vi "Start Point.vi"(5 "Series Enqueuer":refnum<class "Message Enqueuer.lvclass">, 7 "Task-Point Ident":string, 8 "error in":errorcluster, 11 "MSS in":refnum<class "MSS.lvclass">) -> (0 "error out":errorcluster, 3 "MSS out":refnum<class "MSS.lvclass">)   [LabVIEW 2023, in "HAL.lvlib" / "MSS.lvclass"]
uses:
  MSS.lvclass
  <vilib>/ActorFramework/Message Enqueuer/Message Enqueuer.lvclass
  MSS.lvclass/MSS.ctl
  MAL/Series/ISeries Actor/ISeries Actor Messages/Log Event Msg/Log Event Msg.lvclass/Log Event Msg.ctl
  <vilib>/ActorFramework/Message Enqueuer/Message Enqueuer.lvclass/Message Enqueuer.ctl
  MAL/Series/ISeries Actor/ISeries Actor Messages/Start Point on Target Msg/Start Point on Target Msg.lvclass/Start Point on Target Msg.ctl
  <vilib>/ActorFramework/Message Enqueuer/Enqueue.vi
  MAL/Series/ISeries Actor/ISeries Actor Messages/Log Event Msg/Log Event Msg.lvclass
  MAL/Series/ISeries Actor/ISeries Actor Messages/Start Point on Target Msg/Start Point on Target Msg.lvclass
  <vilib>/Utility/LVClass/Get LV Class Name.vi
  <resource>/AFDebug/Generate Trace for Message.vi
  <vilib>/ActorFramework/Message Priority Queue/Priority Enqueue.vi
  Virtual Instruments/Virtual Instrument/Virtual Instrument.lvclass
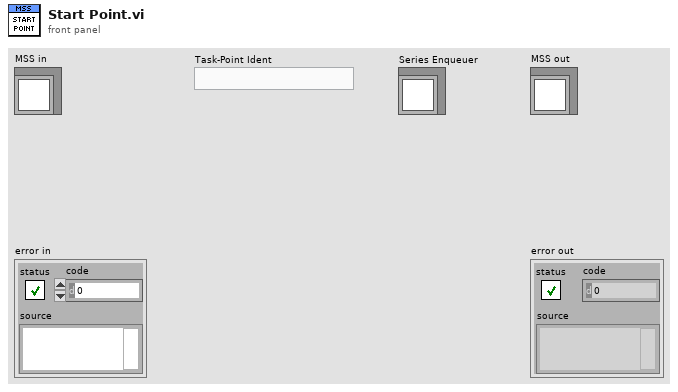
[diagram p1: front panel]
types:
  T1 = map{string, refnum<class "Virtual Instrument.lvclass">}
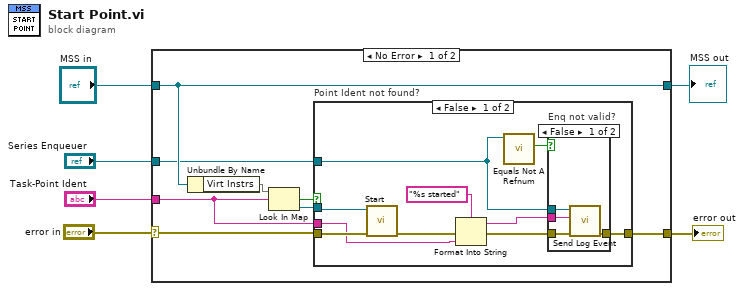
[diagram p0: block diagram]
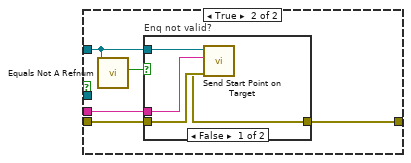
[diagram p3: hidden frame]
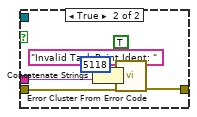
[diagram p4: hidden frame]
diagram:
  n1 = case shown="No Error" "error in" {
    selector: "error in" -> [w10 w47]
    tunnel: [w14 w47] -> w6
    tunnel: "MSS in" -> [w9 w46]
    tunnel: "Task-Point Ident" -> [w8 _]
    tunnel: [w9 w46] -> w3
    tunnel: "Series Enqueuer" -> [w7 _]
    frame No Error {
      n2 = Unbundle By Name(w9) -> ("Virt Instrs"=w13:T1)
      n3 = Look In Map(map=w13, key=w8) -> (key not found?=w11:bool, value=w12:refnum<class "Virtual Instrument.lvclass">)  [unwired: 1 in]
      n4 = case "Point Ident not found?" shown="False" w11 {
        tunnel: w12 -> [w23 _]
        tunnel: w10 -> [w24 w33]
        tunnel: [w17 w34] -> w14
        tunnel: w8 -> [w19 w32]
        tunnel: w7 -> [w15 w30]
        frame False {
          n5 = call "Start.vi"("error in"=w24, "Virtual Instrument in"=w23) -> ("error out"=w22:errorcluster)  [unwired: 8 in, 1 out]
          n6 = Format Into String(format string="%s started", error in=w22, w19) -> (resulting string=w20:string, error out=w18:errorcluster)  [unwired: 1 in]
          n7 = call <vilib>:"Equals Not A Refnum.vi"("Message Enqueuer"=w15) -> ("Not a refnum?"=w16:bool)  [unwired: 10 in]
          n8 = case "Enq not valid?" shown="False" w16 {
            tunnel: w15 -> [w28 _]
            tunnel: w20 -> [w27 _]
            tunnel: w18 -> [w26 w29]
            tunnel: [w25 w29] -> w17
            frame False {
              n9 = call "Send Log Event.vi"("error in (no error)"=w26, "Event Text"=w27, "Message Enqueuer"=w28) -> ("error out"=w25:errorcluster)  [unwired: 7 in, 1 out]
            }
            frame True {
            }
          }
        }
        frame True {
          n10 = call <vilib>:"Equals Not A Refnum.vi"("Message Enqueuer"=w30) -> ("Not a refnum?"=w31:bool)  [unwired: 10 in]
          n11 = case "Enq not valid?" shown="False" w31 {
            tunnel: [w35 w39] -> w34
            tunnel: w33 -> [w37 w40]
            tunnel: w32 -> [w36 w42]
            tunnel: w30 -> [w38 _]
            frame False {
              n12 = call "Send Start Point on Target.vi"("error in (no error)"=w37, "Point Ident"=w36, "Message Enqueuer"=w38) -> ("error out"=w35:errorcluster)  [unwired: 7 in, 1 out]
            }
            frame True {
              n13 = Concatenate Strings("Invalid Task-Point Ident: ", w42) -> (w43:string)
              n14 = call <vilib>:"Error Cluster From Error Code.vi"("show call chain? (False)"=TRUE, "error in (no error)"=w40, "error message (\"\")"=w43, "error code (0)"=5118) -> ("error out"=w39:errorcluster)  [unwired: 5 in]
            }
          }
        }
      }
    }
    frame Error {
    }
  }
  "error out" <- w6
  "MSS out" <- w3
